vi "Hide window.vi"(8 "error in (no error)":errorcluster, 11 "LV MDI in":refnum<class "LV MDI.lvclass">) -> (0 "error out":errorcluster, 3 "LV MDI out":refnum<class "LV MDI.lvclass">)   [LabVIEW 2016, in "LV MDI.lvclass"]
doc: "Hides the window."
uses:
  LV MDI.lvclass
  LV MDI.lvclass/LV MDI.ctl
  user32.dll
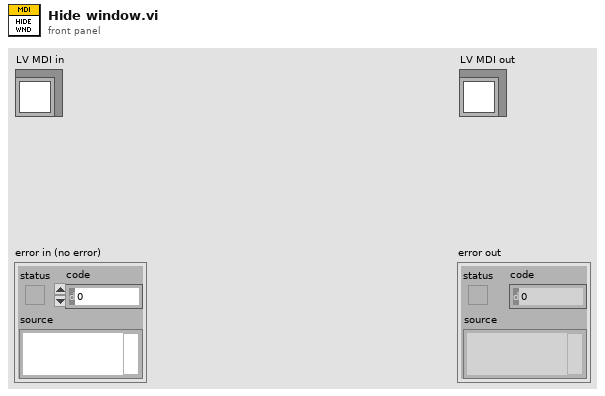
[diagram p1: front panel]
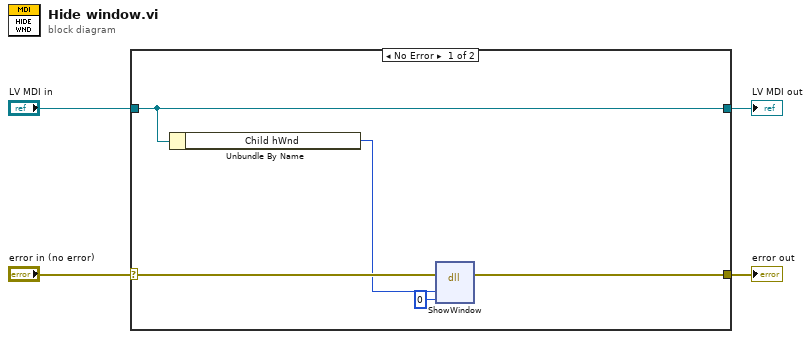
[diagram p0: block diagram]
diagram:
  n1 = case shown="No Error" "error in (no error)" {
    selector: "error in (no error)" -> [w9 w11]
    tunnel: [w6 w11] -> w3
    tunnel: [w5 w10] -> w1
    tunnel: "LV MDI in" -> [w5 w10]
    frame No Error {
      n2 = Unbundle By Name(w5) -> ("Child hWnd"=w8:u32)
      n3 = dll-call lib="user32.dll" fn="ShowWindow"(error in=w9, "hwnd"=w8, "nCmdShow"=u32 0) -> (error out=w6:errorcluster)  [unwired: 5 in, 1 out]
    }
    frame Error {
    }
  }
  "error out" <- w3
  "LV MDI out" <- w1
